vi "Main.vi"() -> ()   [LabVIEW 2018, in "Module A.lvlib"]
uses:
  Module A.lvlib
  Private/ctl/Message Data--cluster.ctl
  Private/ctl/State--enum.ctl
  Common/Common.lvlib
  Module B/Module B.lvlib
panel:
  in  "Start Module B":bool
  out "Msg":string
  in  "Shut Module B":bool
  out "error out":errorcluster
  in  "Error in":errorcluster
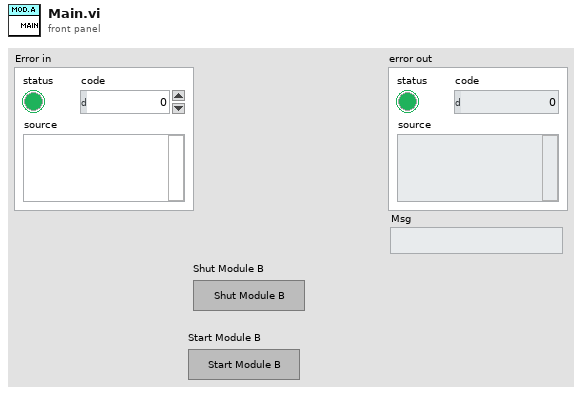
[diagram p1: front panel]
types:
  T1 = typedef "Module A.lvlib/Message Data--cluster.ctl" = cluster{"State":T2, "Data":variant}
  T2 = typedef "Module A.lvlib/State--enum.ctl" = enum16{"Initialize", "Error", "Shut Down", "Stop Module", "---", "Template", "Shut Module B", "Start Module B"}
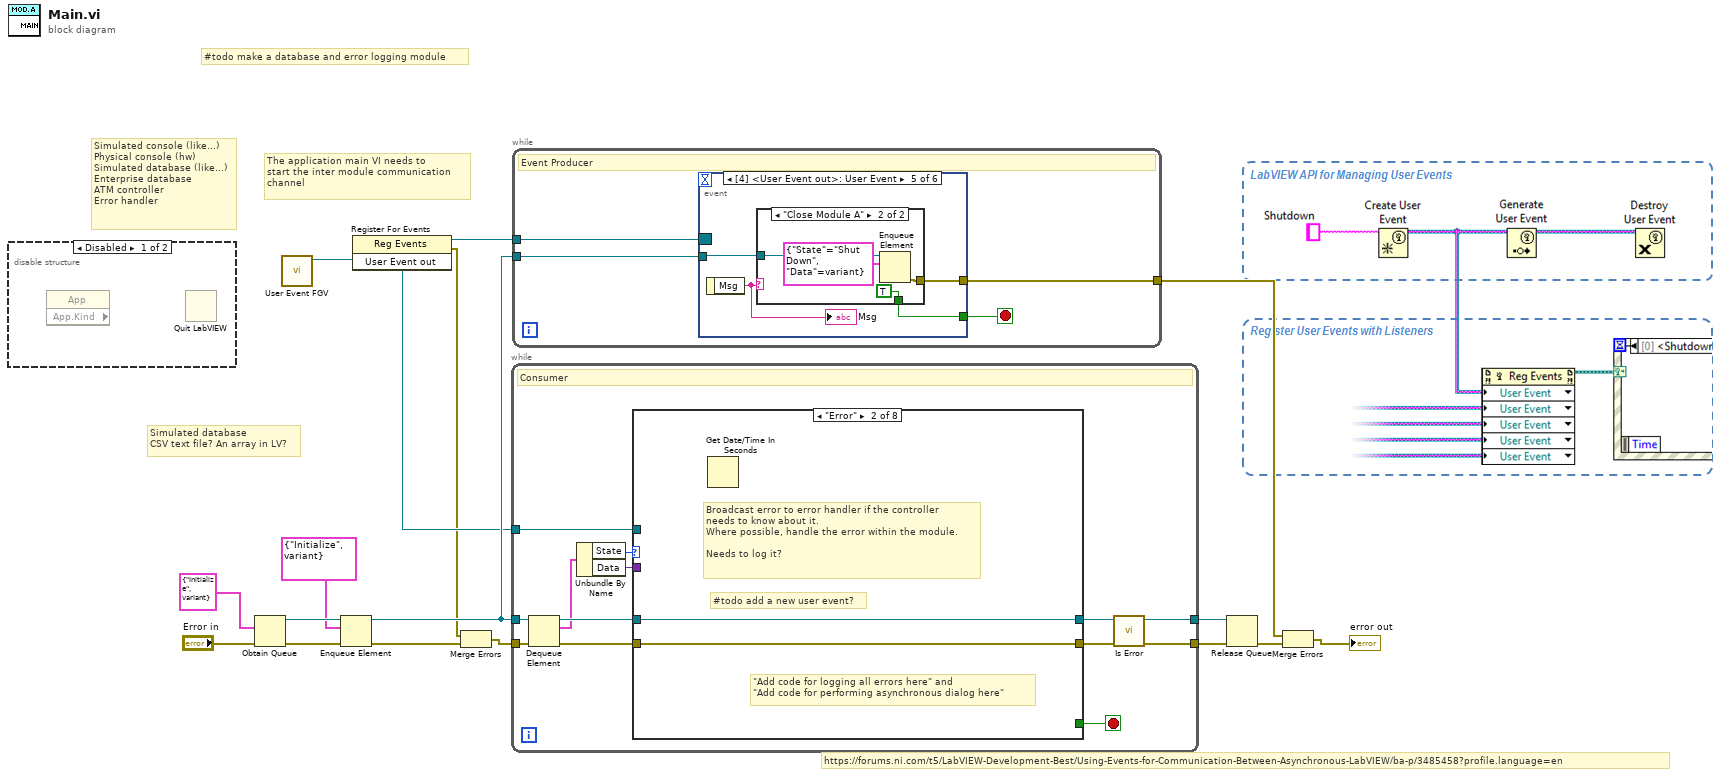
[diagram p0: block diagram]
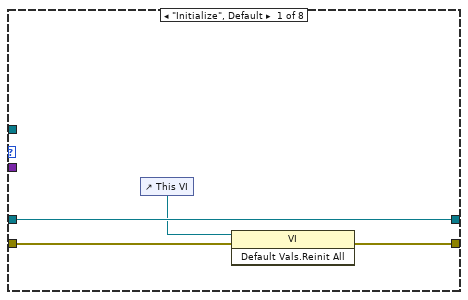
[diagram p3: hidden frame]
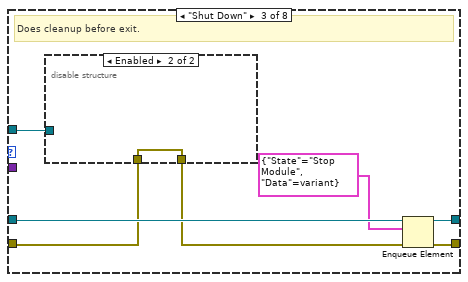
[diagram p4: hidden frame]
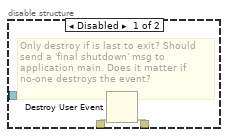
[diagram p5: hidden frame]
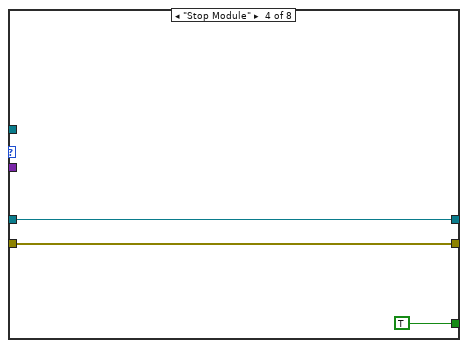
[diagram p6: hidden frame]
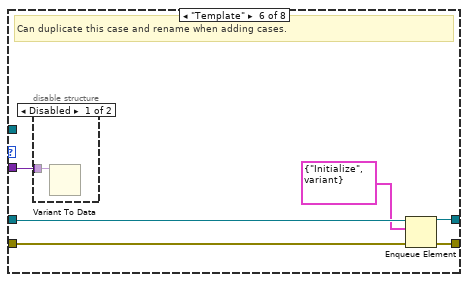
[diagram p8: hidden frame]
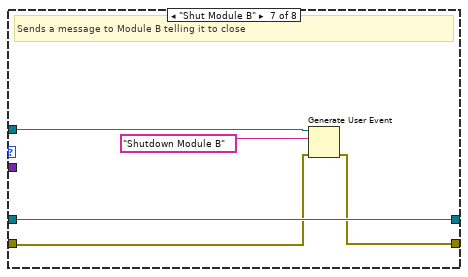
[diagram p10: hidden frame]
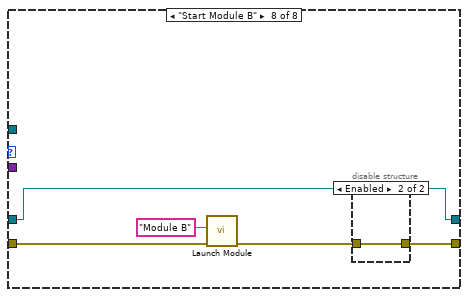
[diagram p11: hidden frame]
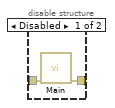
[diagram p12: hidden frame]
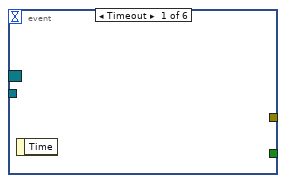
[diagram p13: hidden frame]
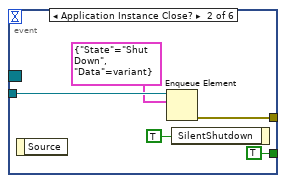
[diagram p14: hidden frame]
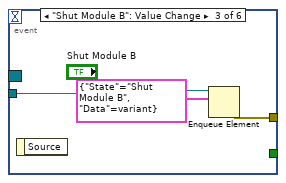
[diagram p15: hidden frame]
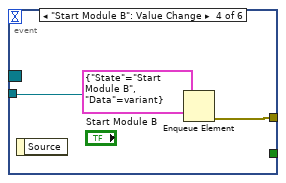
[diagram p16: hidden frame]
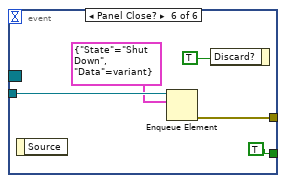
[diagram p18: hidden frame]
diagram:
  # "#todo make a database and error logging module"
  # "The application main VI needs to\nstart the inter module communication\nchannel"
  # "https://forums.ni.com/t5/LabVIEW-Development-Best/Using-Events-for-Communication-Between-Asynchronous-LabVIEW/ba-p/3485458?profile.language=en"
  # "Simulated database\nCSV text file? An array in LV?"
  # "Simulated console (like...)\nPhysical console (hw)\nSimulated database (like...)\nEnterprise database \nATM controller\nError handler"
  n1 = disable-structure shown="Disabled" {
    frame Disabled {
      n2 = property class="App" props=["App.Kind"]() -> ()  [unwired: 2 in, 3 out]
      n3 = Quit LabVIEW() -> ()  [unwired: 1 in]
    }
    frame Enabled {
    }
  }
  n4 = Obtain Queue(element data type=T1 {"State"=enum."Initialize", "Data"=variant} ("Message Data--cluster"), error in (no error)="Error in") -> (queue out=w12:refnum<queue>, error out=w16:errorcluster)  [unwired: 3 in, 1 out]
  n5 = call "User Event FGV.vi"() -> ("User Event out"=w4:refnum<user-event>)  [unwired: 11 in]
  n6 = Enqueue Element(queue=w12, element=T1 {"State"=enum."Initialize", "Data"=variant}, error in (no error)=w16) -> (queue out=w11:refnum<queue>, error out=w2:errorcluster)  [unwired: 1 in, 1 out]
  n7 = register-events(w4) -> (reference out=w5:refnum<event-registration>, error out=w1:errorcluster)  [unwired: 2 in]
  n8 = Merge Errors(w1, w2) -> (w3:errorcluster)
  n9 = while {
    tunnel: w11 -> [w29]
    tunnel: w3 -> [w28]
    tunnel: [w20] -> w14
    tunnel: [w21] -> w13
    tunnel: w4 -> [w17]
    stop <- w18 stop-if-true
    # "Consumer"
    n10 = Dequeue Element(queue=w29, error in (no error)=w28) -> (queue out=w27:refnum<queue>, element=w26:T1, error out=w24:errorcluster)  [unwired: 1 in, 1 out]
    n11 = Unbundle By Name(w26) -> ("State"=w25:T2, "Data"=w23:variant)
    n12 = case shown="\"Error\"" w25 {
      tunnel: w27 -> [w33 w35 w42 w48 w51 w54 w63 w67]
      tunnel: [w33 w35 w41 w48 w51 w55 w63 w67] -> w19
      tunnel: w24 -> [w30 w34 w38 w47 w50 w53 w60 w65]
      tunnel: [w31 w34 w40 w47 w50 w56 w61 w68] -> w22
      tunnel: w23 -> [_ _ _ _ _ w57 _ _]
      tunnel: [_ _ _ TRUE _ _ _ _] -> w18
      tunnel: w17 -> [_ _ w36 _ _ _ w59 _]
      frame "Initialize", Default {
        n13 = control-ref of="This VI"() -> (w32:refnum<vi>)
        n14 = invoke class="VI" method="Default Vals.Reinit All"(reference=w32, error in=w30) -> (error out=w31:errorcluster)  [unwired: 1 in, 2 out]
      }
      frame "Error" {
        # "#todo add a new user event?"
        # "\"Add code for logging all errors here\" and \n\"Add code for performing asynchronous dialog here\""
        # "Broadcast error to error handler if the controller \nneeds to know about it.\nWhere possible, handle the error within the module.\n\nNeeds to log it?"
        n15 = Get Date/Time In Seconds() -> ()  [unwired: 1 out]
      }
      frame "Shut Down" {
        # "Does cleanup before exit."
        n16 = disable-structure shown="Enabled" {
          disable-tunnel: w38 -> [w45 w46]
          disable-tunnel: [w44 w46] -> w37
          disable-tunnel: w36 -> [w43 _]
          frame Disabled {
            # "Only destroy if is last to exit? Should \nsend a 'final shutdown' msg to \napplication main. Does it matter if \nno-one destroys the event?"
            n17 = Destroy User Event(user event=w43, error in=w45) -> (error out=w44:errorcluster)
          }
          frame Enabled {
          }
        }
        n18 = Enqueue Element(queue=w42, element=T1 {"State"=enum."Stop Module", "Data"=variant}, error in (no error)=w37) -> (queue out=w41:refnum<queue>, error out=w40:errorcluster)  [unwired: 1 in, 1 out]
      }
      frame "Stop Module" {
      }
      frame "---" {
        # "Divider - no code."
      }
      frame "Template" {
        # "Can duplicate this case and rename when adding cases."
        n19 = disable-structure shown="Disabled" {
          disable-tunnel: w57 -> [w58 _]
          frame Disabled {
            n20 = Variant To Data(Variant=w58) -> ()  [unwired: 2 in, 2 out]
          }
          frame Enabled {
          }
        }
        n21 = Enqueue Element(queue=w54, element=T1 {"State"=enum."Initialize", "Data"=variant}, error in (no error)=w53) -> (queue out=w55:refnum<queue>, error out=w56:errorcluster)  [unwired: 1 in, 1 out]
      }
      frame "Shut Module B" {
        # "Sends a message to Module B telling it to close"
        n22 = Generate User Event(user event=w59, event data cluster="Shutdown Module B" ("event data"), error in=w60) -> (error out=w61:errorcluster)  [unwired: 1 in, 1 out]
      }
      frame "Start Module B" {
        n23 = call "Launch Module.vi"("error in (no error)"=w65, "Module Name"="Module B") -> ("error out"=w66:errorcluster)  [unwired: 9 in]
        n24 = disable-structure shown="Enabled" {
          disable-tunnel: [w70 w71] -> w68
          disable-tunnel: w66 -> [w69 w71]
          frame Disabled {
            n25 = call "Main.vi"("Error in"=w69) -> ("error out"=w70:errorcluster)  [unwired: 10 in]
          }
          frame Enabled {
          }
        }
      }
    }
    n26 = call "Is Error.vi"("error in"=w22, "Queue in"=w19) -> ("error out"=w21:errorcluster, "Queue out"=w20:refnum<queue>)  [unwired: 8 in]
  }
  n27 = while {
    tunnel: w11 -> [w75]
    tunnel: [w74] -> w6
    tunnel: w5 -> [w72]
    stop <- w73 stop-if-true
    # "Event Producer"
    n28 = event shown="[4] <User Event out>: User Event" {
      selector: w72 -> [_ _ _ _ _ _]
      dyn-events: _ -> [_ _ _ _ _ _]
      timeout: _ -> [_ _ _ _ _ _]
      tunnel: w75 -> [_ w78 w83 w85 w87 w97]
      tunnel: [_ w79 w82 w86 w89 w98] -> w74
      tunnel: [_ TRUE _ _ w88 TRUE] -> w73
      event Timeout {
        n29 = event-data() -> ()  [unwired: 1 in, 1 out]
      }
      event Application Instance Close? {
        n30 = event-data() -> ()  [unwired: 1 in, 1 out]
        n31 = Enqueue Element(queue=w78, element=T1 {"State"=enum."Shut Down", "Data"=variant}) -> (error out=w79:errorcluster)  [unwired: 2 in, 2 out]
        n32 = event-data("SilentShutdown"=TRUE) -> ()  [unwired: 1 in, 1 out]
      }
      event "Shut Module B": Value Change {
        n33 = event-data() -> ()  [unwired: 1 in, 1 out]
        n34 = Enqueue Element(queue=w83, element=T1 {"State"=enum."Shut Module B", "Data"=variant}) -> (error out=w82:errorcluster)  [unwired: 2 in, 2 out]
      }
      event "Start Module B": Value Change {
        n35 = event-data() -> ()  [unwired: 1 in, 1 out]
        n36 = Enqueue Element(queue=w85, element=T1 {"State"=enum."Start Module B", "Data"=variant}) -> (error out=w86:errorcluster)  [unwired: 2 in, 2 out]
      }
      event User Event {
        n37 = event-data() -> ("Msg"=w90:string)  [unwired: 1 in]
        "Msg" <- w90
        n38 = case shown="\"Close Module A\"" w90 {
          tunnel: [_ w94] -> w89
          tunnel: [_ TRUE] -> w88
          tunnel: w87 -> [_ w92]
          frame "False", Default {
          }
          frame "Close Module A" {
            n39 = Enqueue Element(queue=w92, element=T1 {"State"=enum."Shut Down", "Data"=variant}) -> (error out=w94:errorcluster)  [unwired: 2 in, 2 out]
          }
        }
      }
      event Panel Close? {
        n40 = event-data() -> ()  [unwired: 1 in, 1 out]
        n41 = Enqueue Element(queue=w97, element=T1 {"State"=enum."Shut Down", "Data"=variant}) -> (error out=w98:errorcluster)  [unwired: 2 in, 2 out]
        n42 = event-data("Discard?"=TRUE ("SilentShutdown")) -> ()  [unwired: 1 in, 1 out]
      }
    }
  }
  n43 = Release Queue(queue=w14, error in (no error)=w13) -> (error out=w7:errorcluster)  [unwired: 1 in, 2 out]
  n44 = Merge Errors(w6, w7) -> (→"error out":errorcluster)
